vi "set_calibration.vi"(5 "y unit":T1, 7 "x unit":T1, 8 "error in (no error)":errorcluster, 9 "y":dbl, 10 "x":dbl, 11 "Image in":refnum<class "Image.lvclass">) -> (0 "error out":errorcluster, 3 "Image out":refnum<class "Image.lvclass">)   [LabVIEW 2010, in "Image.lvclass"]
uses:
  Image.lvclass
  enumerations/unit.ctl
  Image.lvclass/Image.ctl
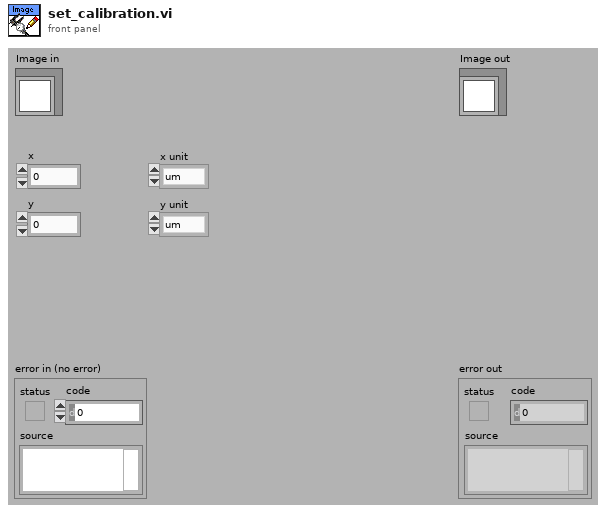
[diagram p1: front panel]
types:
  T1 = typedef "Image.lvclass/unit.ctl" = enum16{"um", "s"}
  T2 = typedef "Image.lvclass/storage_mode.ctl" = enum16{"RAM", "disk"}
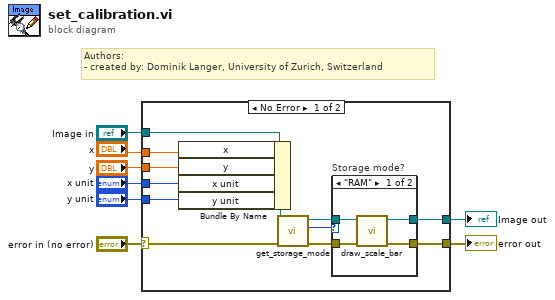
[diagram p0: block diagram]
diagram:
  # "Authors: \n- created by: Dominik Langer, University of Zurich, Switzerland"
  n1 = case shown="No Error" "error in (no error)" {
    selector: "error in (no error)" -> [w15 w28]
    tunnel: [w17 w28] -> w7
    tunnel: [w16 w27] -> w5
    tunnel: "Image in" -> [w18 w27]
    tunnel: "x" -> [w20 _]
    tunnel: "y" -> [w19 _]
    tunnel: "x unit" -> [w10 _]
    tunnel: "y unit" -> [w9 _]
    frame No Error {
      n2 = Bundle By Name(cluster=w18, "x"=w20, "y"=w19, "x unit"=w10, "y unit"=w9) -> (w12:refnum<class "Image.lvclass">)
      n3 = call-dynamic "get_storage_mode.vi"("error in (no error)"=w15, "Image.lvclass in"=w12) -> ("error out"=w14:errorcluster, "storage mode"=w11:T2, "Image.lvclass out"=w13:refnum<class "Image.lvclass">)  [unwired: 7 out]
      n4 = case "Storage mode?" shown="\"RAM\"" w11 {
        tunnel: w14 -> [w21 w25]
        tunnel: w13 -> [w22 w26]
        tunnel: [w24 w25] -> w17
        tunnel: [w23 w26] -> w16
        frame "RAM" {
          n5 = call "draw_scale_bar.vi"("error in (no error)"=w21, "Image in"=w22) -> ("error out"=w24:errorcluster, "Image out"=w23:refnum<class "Image.lvclass">)  [unwired: 3 in, 5 out]
        }
        frame "disk", Default {
        }
      }
    }
    frame Error {
    }
  }
  "error out" <- w7
  "Image out" <- w5
